vi "FPGAmain_5160.vi"() -> ()   [LabVIEW 2013]
uses:
  FPGA/DataMode.ctl
  FPGA/AcquireState.ctl
  <vilib>/Platform/TimedLoop/XDataNode/timing_clust.ctl
  <vilib>/Platform/TimedLoop/XDataNode/nitl_modes.ctl
  <vilib>/Platform/TimedLoop/XDataNode/wakeup.ctl
  <vilib>/rvi/Emulation/niFpgaSctlEmulationGetInTimedLoop.vi
  <vilib>/rvi/Emulation/niFpgaEmulationReportErrorSimple.vi
  <vilib>/rvi/Emulation/niFpgaGetClockAttributes.vi
  <vilib>/rvi/eio/common/nirviEmuTemplateMethod_errors.vi
  <vilib>/rvi/Emulation/niFpgaCriticalErrorInLSC.vi
  <vilib>/rvi/FIFO/Fifo_Resource/nirvififoEmulationWriteFpgaImpl.vi
  <vilib>/rvi/DataTransferAndStorage/Container/Common/niFpgaContainerGetUniqueNameForEmu.vi
  <vilib>/rvi/FIFO/Fifo_Resource/nirvififoEmulationReadFpgaImpl.vi
  <vilib>/rvi/DataTransferAndStorage/Register/Emulation/niFpgaRegisterEmulationFpgaImpl.vi
  <instcachedir>/0/niFpgaRegisterEmulationFpgaImpl_DCF4BC0110594B98B44A971D60CEEC4D.lvgen/niFpgaRegisterEmulationFpgaImpl_DCF4BC0110594B98B44A971D60CEEC4D_016.vi
  <instcachedir>/0/niFpgaRegisterEmulationFpgaImpl_DCF4BC0110594B98B44A971D60CEEC4D.lvgen/niFpgaRegisterEmulationFpgaImpl_DCF4BC0110594B98B44A971D60CEEC4D_003.vi
  <instcachedir>/0/niFpgaRegisterEmulationFpgaImpl_DCF4BC0110594B98B44A971D60CEEC4D.lvgen/niFpgaRegisterEmulationFpgaImpl_DCF4BC0110594B98B44A971D60CEEC4D_014.vi
  <instcachedir>/0/niFpgaRegisterEmulationFpgaImpl_DCF4BC0110594B98B44A971D60CEEC4D.lvgen/niFpgaRegisterEmulationFpgaImpl_DCF4BC0110594B98B44A971D60CEEC4D_015.vi
  <vilib>/rvi/interface/RandomDataEmulation/nirviRandomDataMultiElementFPGAFIFO.vi
  <instcachedir>/0/nirviRandomDataMultiElementFPGAFIFO_F2B80EDE0D7944A08478D8D26097D4DB.lvgen/nirviRandomDataMultiElementFPGAFIFO_F2B80EDE0D7944A08478D8D26097D4DB_005.vi
  <vilib>/rvi/interface/RandomDataEmulation/niFpgaRandomDataHandleErrors.vi
  <vilib>/rvi/interface/RandomDataEmulation/nirviRandomDataFPGAFIFO.vi
  <vilib>/Platform/TimedLoop/XDataNode/XDataNode.xnode
  <vilib>/eio/EIONode/EIONode.xnode
  <vilib>/rvi/DataTransferAndStorage/Container/XNode/niFpgaContainer.xnode
  <vilib>/rvi/FIFO/Fifo_Resource/nirvififoEmulationWrite.vi
  <vilib>/rvi/FIFO/Fifo_Resource/nirvififoEmulationRead.vi
  <vilib>/rvi/DataTransferAndStorage/Register/Emulation/niFpgaRegisterEmulation.vi
  <vilib>/rvi/interface/RandomDataEmulation/nirviRandomDataFpgaMultiElementTemplate.vi
  <vilib>/rvi/interface/RandomDataEmulation/nirviRandomDataFpgaReadWriteTemplate.vi
  <vilib>/rvi/FIFO/Fifo_Resource/nirvififoEmulationP2P.vi
  <vilib>/Platform/TimedLoop/XDataNode/XDNodeRunTimeDep.lvlib
  <instrlib>/FlexRIO/Libraries/Helper VIs/NI FlexRIO Helper VIs.lvlib
  FPGA/Input_5782/5782_states.ctl
panel:
  in  "delay phase":fxp<+,64,64>
  in  "AM phase":fxp<+,64,64>
  in  "Phase 5782":fxp<+,64,64>[](array[numeric])=[0.0, 0.0]
  in  "User Command Commit":bool
  in  "User Command":u8
  out "User Command Idle":bool
  out "User Command Status":u8
  in  "User Data 0":u8
  in  "User Data 1":u8
  out "PLL Locked":bool
  out "User Error":bool
  out "Configured?":bool
  in  "FIR coeffs":fxp<+/-,18,18>[](array[numeric])
  in  "Phase output":fxp<+,64,64>[](array[numeric])=[0.0, 0.0, 0.0, 0.0]
  in  "5782 record length":u16=4000 caption="Samples Per Trigger" min=1 step=1
  in  "Trigger Acquisition":bool
  in  "Continuous":bool
  out "IO Module\\Trigger Input":bool
  in  "Mode":T1
  in  "Simulated phase 5782":fxp<+,64,64>[](array[numeric])=[0.0, 0.0]
  in  "Acquisition running":bool
  in  "Samples Per Trigger":i32 min=1 step=1
  in  "Trigger simulated data":bool
  in  "simulated phase 5160":fxp<+,64,64>
  in  "phase 5160":fxp<+,64,64>
  # "Dynamic filter"
  # "Dynamic downsample"
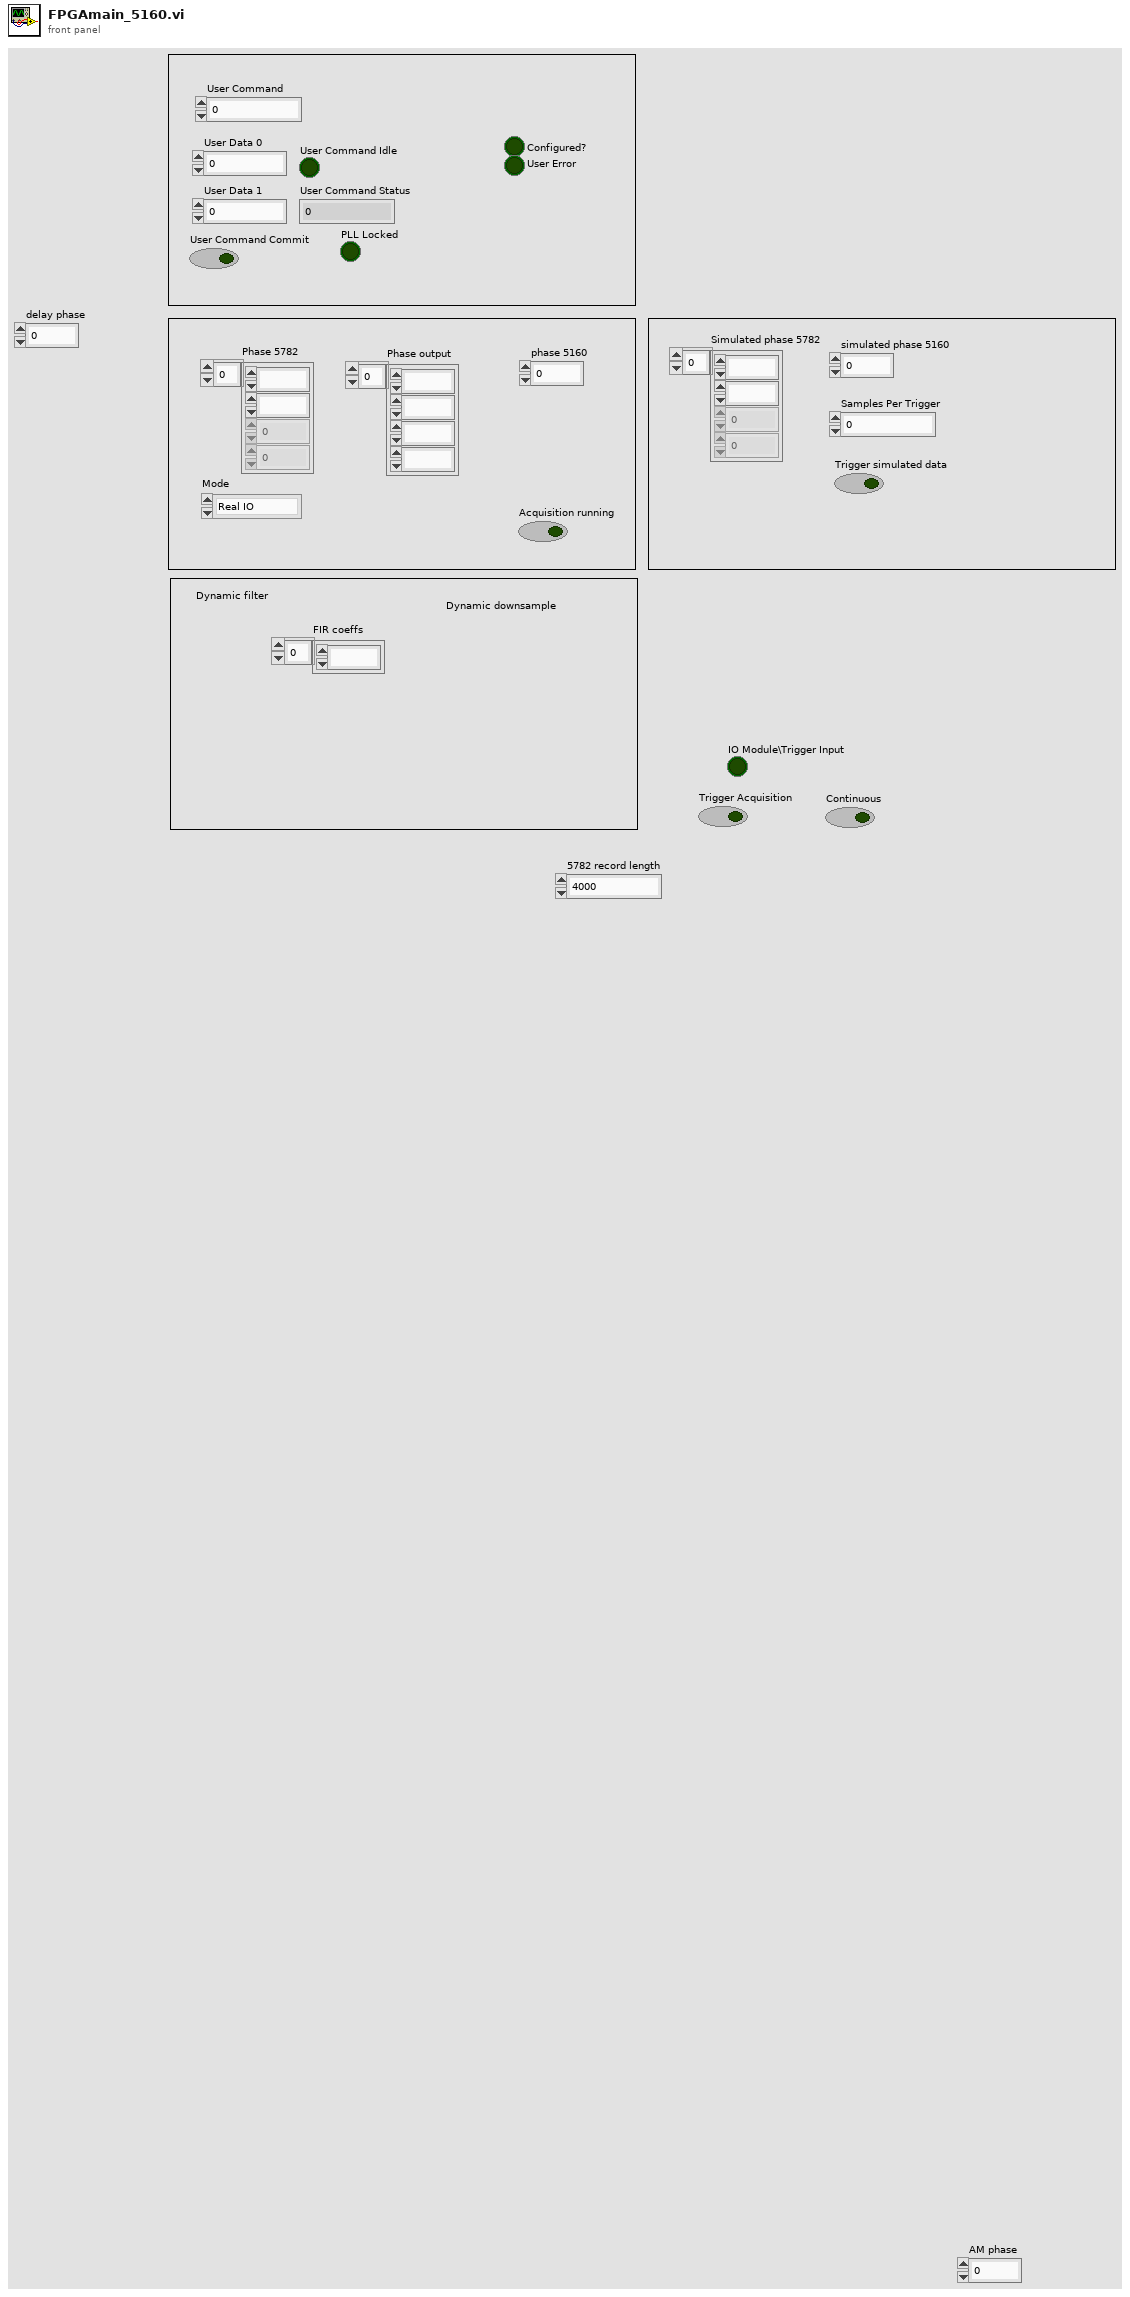
[diagram p1: front panel]
types:
  T1 = typedef "DataMode.ctl" = enum16{"Real IO", "Simulated"}
  T2 = typedef "AcquireState.ctl" = enum8{"Idle", "Acquire"}
  T3 = typedef "5782_states.ctl" = enum8{"Wait for trigger", "Acquisition", "Send record length", "Quiet period"}
  T4 = typedef "XDNodeRunTimeDep.lvlib/timing_clust.ctl" = cluster{"Expected End [f-1]":u64, "Actual End [f-1]":u64, "Finished Late? [f-1]":bool, "Expected End [i-1]":u64, "Actual End [i-1]":u64, "Finished Late? [i-1]":bool, "Expected Start [i]":u64, "Actual Start [i]":u64, "Expected Start [f]":u64, "Actual Start [f]":u64, "Source Name":string, "Structure Name":string, "Period":i64, "Deadline":i64, "Offset":i64, "Start":i64, "Priority":i32, "Timeout":i32, "Mode":T5, "Wakeup Reason":T6, "Error":errorcluster, "Source Type":string, "Secondary Source Type":string, "Global End Time":u64, "Global Start Time":u64, "Frame Duration":u64, "Iteration Duration":u64, "Assigned CPU":i32, "I/O Scan Engine Mode":u32}
  T5 = typedef "XDNodeRunTimeDep.lvlib/nitl_modes.ctl" = enum32{"No Change", "Process missed periods, maintain original phase", "Discard missed periods, maintain original phase", "Process missed periods, ignore original phase", "Discard missed periods, ignore original phase"}
  T6 = typedef "XDNodeRunTimeDep.lvlib/wakeup.ctl" = enum32{"Normal", "Aborted", "Asynchronous wakeup", "Timing source error", "Timed loop error", "Timeout"}
  T7 = typedef "I16 array size 2.ctl" = i16[]
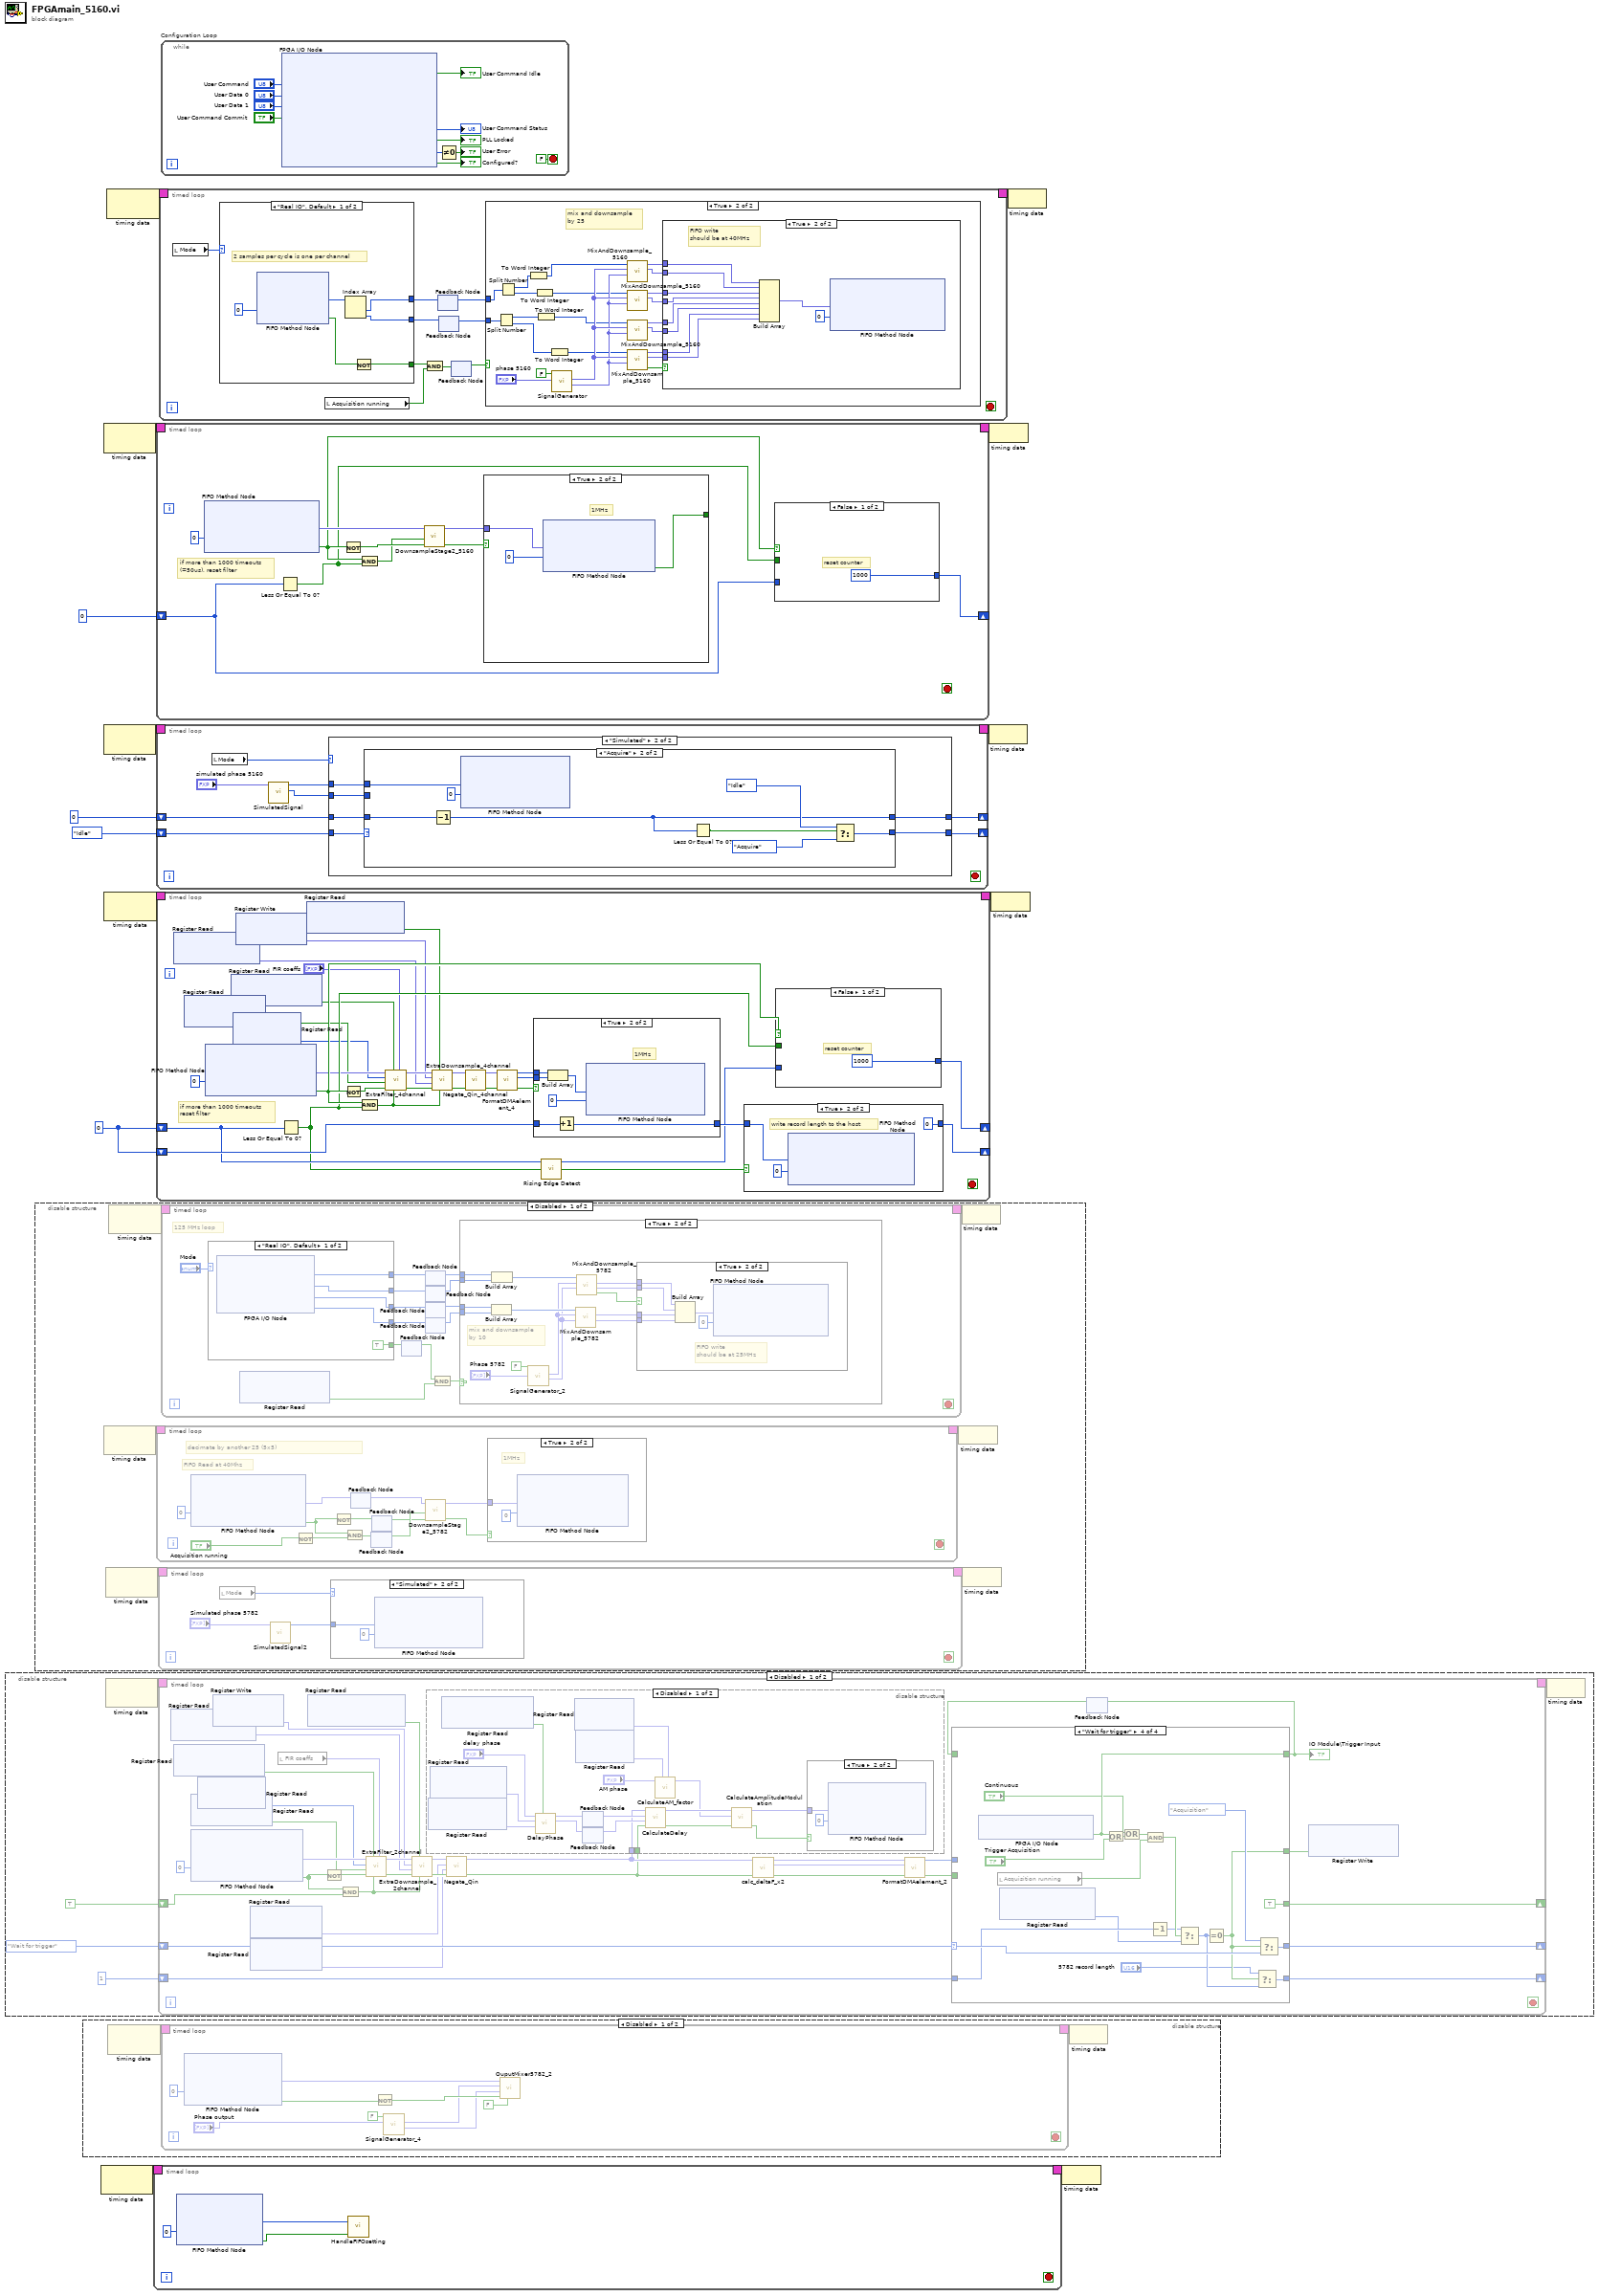
[diagram p0: block diagram]
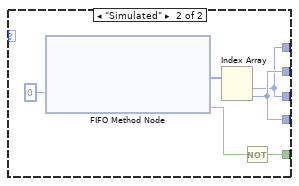
[diagram p4: hidden frame]
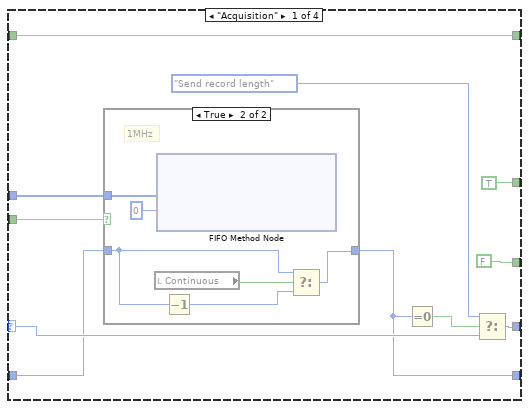
[diagram p10: hidden frame]
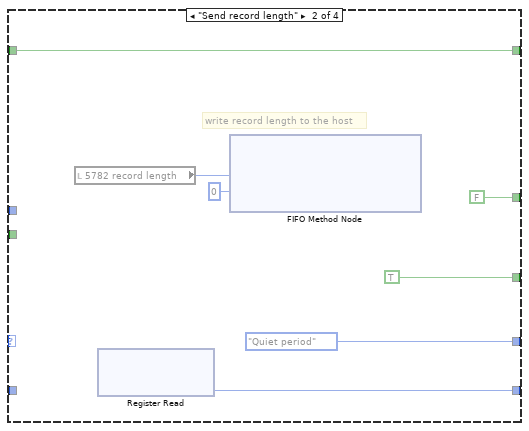
[diagram p12: hidden frame]
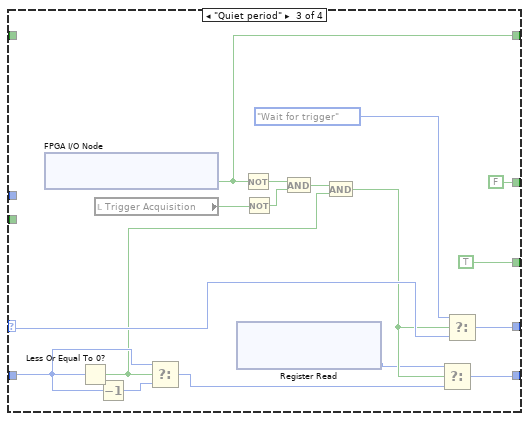
[diagram p13: hidden frame]
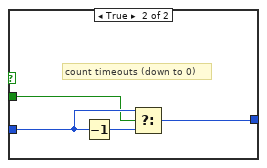
[diagram p16: hidden frame]
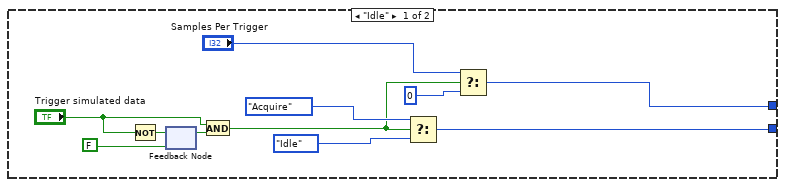
[diagram p20: hidden frame]
diagram:
  w3 = 0 ("y")
  n1 = disable-structure shown="Disabled" {
    frame Disabled {
      n2 = node-c288() -> (w19:T4)  [unwired: 1 in]
      n3 = timed-loop {
        timing: w19 -> [_]
        timing-out: [_] -> w18
        shift-right: [w51] -> _
        shift-left: 5782_states."Wait for trigger" ("5782 states") -> [w53]
        shift-right: [w50] -> _
        shift-left: u16 1 ("trigger samples") -> [w52]
        shift-right: [w39] -> _
        shift-left: TRUE -> [w42]
        stop <- _ stop-if-true
        n4 = xnode ("Register Read")() -> ("Data"=w24:fxp<+,8,8>)  [unwired: 1 in, 1 out]
        n5 = xnode ("Register Read")() -> ("Data"=w30:bool)  [unwired: 1 in, 1 out]
        n6 = xnode ("Register Read")() -> ("Data"=w25:bool)  [unwired: 1 in, 1 out]
        n7 = xnode ("FIFO Method Node")("Timeout"=0) -> ("Element"=w44:fxp<+/-,16,14>[], "Timed Out?"=w43:bool)  [unwired: 1 in, 1 out]
        n8 = xnode ("Register Read")() -> ("Data"=w26:i32)  [unwired: 1 in, 1 out]
        n9 = xnode ("Register Write")() -> ("Data"=w23:fxp<+/-,32,1>)  [unwired: 1 in, 1 out]
        n10 = xnode ("Register Read")() -> ("Data"=w28:fxp<+/-,16,14>)  [unwired: 1 in, 1 out]
        n11 = xnode ("Register Read")() -> ("Data"=w29:fxp<+/-,16,14>)  [unwired: 1 in, 1 out]
        n12 = local read "FIR coeffs"() -> (w22:fxp<+/-,18,18>[])
        n13 = xnode ("Register Read")() -> ("Data"=w27:bool)  [unwired: 1 in, 1 out]
        n14 = Not(x=w43) -> (.not. x?=w46:bool)
        n15 = And(x=w43, y=w42) -> (x .and. y?=w48:bool)
        n16 = call "ExtraFilter_2channel.vi"(5:"new coeffs"=w22, "reset"=w48, 7:"new coeffs"=w30, "valid in"=w46, "enable filter"=w25, "new shift"=w26, "Data in"=w44) -> ("valid out"=w47:bool, "Data out"=w45:fxp<+/-,16,14>[])  [unwired: 3 in]
        n17 = call "ExtraDownsample_2channel.vi"("reset"=w48, "Set downsample"=w27, "valid in"=w47, "Downsample"=w24, "CIC Gain"=w23, "Data in"=w45) -> ("valid out"=w36:bool, "Data out"=w37:fxp<+/-,16,14>[])  [unwired: 4 in]
        n18 = call "Negate_Qin.vi"("valid in"=w36, "DC offset chan 1"=w28, "DC offset chan 0"=w29, "Data in"=w37) -> ("valid out"=w33:bool, "Data out"=w35:fxp<+/-,16,14>[])  [unwired: 6 in]
        n19 = disable-structure shown="Disabled" {
          disable-tunnel: w35 -> [w64 _]
          disable-tunnel: w33 -> [w60 _]
          frame Disabled {
            n20 = xnode ("Register Read")() -> ("Data"=w55:fxp<+/-,16,0>)  [unwired: 1 in, 1 out]
            n21 = xnode ("Register Read")() -> ("Data"=w56:fxp<+/-,16,0>)  [unwired: 1 in, 1 out]
            n22 = xnode ("Register Read")() -> ("Data"=w57:bool)  [unwired: 1 in, 1 out]
            n23 = call "DelayPhase.vi"("Use fixed delay"=w57, "fixed cos_fi"=w55, "fixed sin fi"=w56, "delay phase"="delay phase") -> ("cos_fi"=w62:fxp<+/-,16,0>, "sin fi"=w63:fxp<+/-,16,0>)  [unwired: 6 in]
            n24 = xnode ("Register Read")() -> ("Data"=w59:fxp<+/-,16,2>)  [unwired: 1 in, 1 out]
            n25 = xnode ("Register Read")() -> ("Data"=w58:fxp<+/-,16,2>)  [unwired: 1 in, 1 out]
            n26 = feedback #1() -> (w71:fxp<+/-,16,0>)  [unwired: 1 in]
            n27 = feedback-in #1(w63) -> ()
            n28 = feedback #2() -> (w70:fxp<+/-,16,0>)  [unwired: 1 in]
            n29 = feedback-in #2(w62) -> ()
            n30 = call "CalculateDelay.vi"("input valid"=w60, "cos_fi"=w70, "sin fi"=w71, "Data in"=w64) -> ("output valid"=w68:bool, "Data out"=w69:fxp<+/-,16,14>[])  [unwired: 6 in]
            n31 = call "CalculateAM_factor.vi"("b_am"=w59, "a_am"=w58, "AM phase"="AM phase") -> ("AM_factor"=w65:fxp<+/-,16,2>)  [unwired: 7 in, 1 out]
            n32 = call "CalculateAmplitudeModulation.vi"("input valid"=w68, "AM_factor"=w65, "Data in"=w69) -> ("output valid"=w66:bool, "Data out"=w67:fxp<+/-,16,14>[])  [unwired: 7 in]
            n33 = case shown="True" w66 {
              tunnel: w67 -> [_ w72]
              frame False {
              }
              frame True {
                n34 = xnode ("FIFO Method Node")("Element"=w72, "Timeout"=0) -> ()  [unwired: 1 in, 2 out]
              }
            }
          }
          frame Enabled {
          }
        }
        n35 = call "calc_deltaF_x2.vi"("valid in"=w33, "Data in"=w35) -> ("valid out"=w32:bool, "deltaF"=w31:fxp<+/-,32,30>[], "Data out"=w34:fxp<+/-,16,14>[])  [unwired: 7 in]
        n36 = call "FormatDMAelement_2.vi"("valid in"=w32, "deltaF"=w31, "Data in"=w34) -> ("valid out"=w40:bool, "Element"=w41:u64[])  [unwired: 7 in]
        n37 = feedback #3() -> (w21:bool)  [unwired: 1 in]
        n38 = case shown="\"Wait for trigger\"" w53 {
          selector: w53 -> [w84 _ w114 w133]
          tunnel: w52 -> [w80 _ w102 w122]
          tunnel: [w83 5782_states."Quiet period" ("5782 states") w113 w132] -> w51
          tunnel: [w77 w92 w115 w131] -> w50
          tunnel: w41 -> [w78 _ _ _]
          tunnel: w40 -> [w79 _ _ _]
          tunnel: [FALSE TRUE TRUE TRUE] -> w39
          tunnel: [TRUE FALSE ("5782 triggered") FALSE ("5782 triggered") w126] -> w38
          tunnel: [w76 w93 w104 w125] -> w20
          tunnel: w21 -> [w76 w93 _ _]
          frame "Acquisition" {
            n39 = case shown="True" w79 {
              tunnel: w78 -> [_ w91]
              tunnel: [w85 w88] -> w77
              tunnel: w80 -> [w85 w86]
              frame False {
              }
              frame True {
                # "1MHz"
                n40 = local read "Continuous"() -> (w89:bool)
                n41 = xnode ("FIFO Method Node")("Element"=w91, "Timeout"=0) -> ()  [unwired: 1 in, 2 out]
                n42 = Decrement(x=w86) -> (x-1=w87:u16)
                n43 = Select(t=w86, s=w89, f=w87) -> (s? t:f=w88:u16)
              }
            }
            n44 = Equal To 0?(x=w77) -> (x = 0?=w81:bool)
            n45 = Select(t=5782_states."Send record length" ("5782 states"), s=w81, f=w84) -> (s? t:f=w83:T3)
          }
          frame "Send record length" {
            # "write record length to the host"
            n46 = local read "5782 record length"() -> (w95:u16)
            n47 = xnode ("Register Read")() -> ("Data"=w92:u16)  [unwired: 1 in, 1 out]
            n48 = xnode ("FIFO Method Node")("Element"=w95, "Timeout"=0) -> ()  [unwired: 1 in, 2 out]
          }
          frame "Quiet period" {
            n49 = xnode "FPGA I/O Node"() -> ("IO Module\\Trigger Input"=w104:bool)  [unwired: 1 in, 1 out]
            n50 = Less Or Equal To 0?(x=w102) -> (x <= 0?=w101:bool)
            n51 = local read "Trigger Acquisition"() -> (w110:bool)
            n52 = Decrement(x=w102) -> (x-1=w103:u16)
            n53 = Select(t=w102, s=w101, f=w103) -> (s? t:f=w100:u16)
            n54 = xnode ("Register Read")() -> ("Data"=w99:u16)  [unwired: 1 in, 1 out]
            n55 = Not(x=w104) -> (.not. x?=w109:bool)
            n56 = Not(x=w110) -> (.not. x?=w108:bool)
            n57 = And(x=w109, y=w108) -> (x .and. y?=w107:bool)
            n58 = And(x=w107, y=w101) -> (x .and. y?=w112:bool)
            n59 = Select(t=w99, s=w112, f=w100) -> (s? t:f=w115:u16)
            n60 = Select(t=5782_states."Wait for trigger" ("5782 states"), s=w112, f=w114) -> (s? t:f=w113:T3)
          }
          frame "Wait for trigger" {
            n61 = xnode "FPGA I/O Node"() -> ("IO Module\\Trigger Input"=w125:bool)  [unwired: 1 in, 1 out]
            n62 = local read "Acquisition running"() -> (w127:bool)
            n63 = xnode ("Register Read")() -> ("Data"=w119:u16)  [unwired: 1 in, 1 out]
            n64 = Or(x=w125, y="Trigger Acquisition") -> (x .or. y?=w121:bool)
            n65 = Or(x="Continuous", y=w121) -> (x .or. y?=w120:bool)
            n66 = And(x=w120, y=w127) -> (x .and. y?=w128:bool)
            n67 = Decrement(x=w122) -> (x-1=w123:u16)
            n68 = Select(t=w123, s=w128, f=w119) -> (s? t:f=w124:u16)
            n69 = Equal To 0?(x=w124) -> (x = 0?=w126:bool)
            n70 = Select(t="5782 record length", s=w126, f=w124) -> (s? t:f=w131:u16)
            n71 = Select(t=5782_states."Acquisition" ("5782 states"), s=w126, f=w133) -> (s? t:f=w132:T3)
          }
        }
        "IO Module\\Trigger Input" <- w20
        n72 = feedback-in #3(w20) -> ()
        n73 = xnode ("Register Write")("Data"=w38) -> ()  [unwired: 1 in, 1 out]
      }
      n74 = node-c288(w18) -> ()
    }
    frame Enabled {
    }
  }
  n75 = disable-structure shown="Disabled" {
    frame Disabled {
      n76 = node-c288() -> (w141:T4)  [unwired: 1 in]
      n77 = node-c288() -> (w143:T4)  [unwired: 1 in]
      n78 = node-c288() -> (w139:T4)  [unwired: 1 in]
      n79 = timed-loop {
        timing: w141 -> [_]
        timing-out: [_] -> w140
        stop <- _ stop-if-true
        # "FIFO Read at 40Mhz"
        # "decimate by another 25 (5x5)"
        n80 = xnode ("FIFO Method Node")("Timeout"=0) -> ("Element"=w199:fxp<+/-,16,14>[], "Timed Out?"=w200:bool)  [unwired: 1 in, 1 out]
        n81 = Not(x="Acquisition running") -> (.not. x?=w201:bool)
        n82 = Not(x=w200) -> (.not. x?=w195:bool)
        n83 = And(x=w200, y=w201) -> (x .and. y?=w197:bool)
        n84 = feedback #4() -> (w198:fxp<+/-,16,14>[])  [unwired: 1 in]
        n85 = feedback-in #4(w199) -> ()
        n86 = feedback #5() -> (w196:bool)  [unwired: 1 in]
        n87 = feedback-in #5(w197) -> ()
        n88 = feedback #6() -> (w194:bool)  [unwired: 1 in]
        n89 = feedback-in #6(w195) -> ()
        n90 = call "DownsampleStage2_5782.vi"("valid in"=w194, "reset"=w196, "Data in"=w198) -> ("valid out"=w202:bool, "data out"=w203:fxp<+/-,16,14>[])  [unwired: 7 in]
        n91 = case shown="True" w202 {
          tunnel: w203 -> [_ w205]
          frame False {
          }
          frame True {
            # "1MHz"
            n92 = xnode ("FIFO Method Node")("Element"=w205, "Timeout"=0) -> ()  [unwired: 1 in, 2 out]
          }
        }
      }
      n93 = timed-loop {
        timing: w143 -> [_]
        timing-out: [_] -> w142
        stop <- _ stop-if-true
        n94 = local read "Mode"() -> (w213:T1)
        n95 = call "SimulatedSignal2.vi"("Phase"="Simulated phase 5782") -> ("output"=w212:T7)  [unwired: 9 in, 1 out]
        n96 = case shown="\"Simulated\"" w213 {
          tunnel: w212 -> [_ w214]
          frame "Real IO", Default {
          }
          frame "Simulated" {
            n97 = xnode ("FIFO Method Node")("Element"=w214, "Timeout"=0) -> ()  [unwired: 1 in, 2 out]
          }
        }
      }
      n98 = timed-loop {
        timing: w139 -> [_]
        timing-out: [_] -> w138
        stop <- _ stop-if-true
        # "125 MHz loop"
        n99 = case shown="\"Real IO\", Default" "Mode" {
          tunnel: [w182 w185] -> w155
          tunnel: [w181 w186] -> w153
          tunnel: [w180 w185] -> w151
          tunnel: [w179 w186] -> w148
          tunnel: [TRUE w183] -> w147
          frame "Real IO", Default {
            n100 = xnode "FPGA I/O Node"() -> ("IO Module\\AI 0 N-1"=w182:i16, "IO Module\\AI 0 N"=w181:i16, "IO Module\\AI 1 N-1"=w180:i16, "IO Module\\AI 1 N"=w179:i16)  [unwired: 4 in, 4 out]
          }
          frame "Simulated" {
            n101 = xnode ("FIFO Method Node")("Timeout"=0) -> ("Element"=w187:i16[], "Timed Out?"=w184:bool)  [unwired: 1 in, 1 out]
            n102 = Index Array(array=w187) -> (element #1=w185:i16, element #2=w186:i16)  [unwired: 2 in]
            n103 = Not(x=w184) -> (.not. x?=w183:bool)
          }
        }
        n104 = xnode ("Register Read")() -> ("Data"=w145:bool)  [unwired: 1 in, 1 out]
        n105 = feedback #7() -> (w146:bool)  [unwired: 1 in]
        n106 = feedback-in #7(w147) -> ()
        n107 = feedback #8() -> (w154:i16)  [unwired: 1 in]
        n108 = feedback-in #8(w155) -> ()
        n109 = feedback #9() -> (w152:i16)  [unwired: 1 in]
        n110 = feedback-in #9(w153) -> ()
        n111 = feedback #10() -> (w150:i16)  [unwired: 1 in]
        n112 = feedback-in #10(w151) -> ()
        n113 = feedback #11() -> (w149:i16)  [unwired: 1 in]
        n114 = feedback-in #11(w148) -> ()
        n115 = And(x=w146, y=w145) -> (x .and. y?=w156:bool)
        n116 = case shown="True" w156 {
          tunnel: w154 -> [_ w162]
          tunnel: w152 -> [_ w161]
          tunnel: w150 -> [_ w160]
          tunnel: w149 -> [_ w159]
          frame False {
          }
          frame True {
            # "mix and downsample\nby 10"
            n117 = Build Array(w160, w159) -> (w171:i16[])
            n118 = Build Array(w162, w161) -> (w158:i16[])
            n119 = call "SignalGenerator_2.vi"("Phase"="Phase 5782", "reset"=FALSE) -> ("Sine out"=w163:fxp<+/-,16,0>[], "Cosine out"=w164:fxp<+/-,16,0>[])  [unwired: 8 in]
            n120 = call "MixAndDownsample_5782.vi"("Sine in"=w163, "Cosine in"=w164, "Signal Input"=w171) -> ("Q out"=w166:fxp<+/-,16,14>, "I out"=w167:fxp<+/-,16,14>)  [unwired: 6 in, 1 out]
            n121 = call "MixAndDownsample_5782.vi"("Sine in"=w163, "Cosine in"=w164, "Signal Input"=w158) -> ("data valid"=w168:bool, "Q out"=w169:fxp<+/-,16,14>, "I out"=w170:fxp<+/-,16,14>)  [unwired: 6 in]
            n122 = case shown="True" w168 {
              tunnel: w169 -> [_ w177]
              tunnel: w170 -> [_ w174]
              tunnel: w167 -> [_ w173]
              tunnel: w166 -> [_ w172]
              frame False {
              }
              frame True {
                # "FIFO write\nshould be at 25MHz"
                n123 = Build Array(w174, w177, w173, w172) -> (w176:fxp<+/-,16,14>[])
                n124 = xnode ("FIFO Method Node")("Element"=w176, "Timeout"=0) -> ()  [unwired: 1 in, 2 out]
              }
            }
          }
        }
      }
      n125 = node-c288(w140) -> ()
      n126 = node-c288(w138) -> ()
      n127 = node-c288(w142) -> ()
    }
    frame Enabled {
    }
  }
  n128 = disable-structure shown="Disabled" {
    frame Disabled {
      n129 = node-c288() -> (w221:T4)  [unwired: 1 in]
      n130 = timed-loop {
        timing: w221 -> [_]
        timing-out: [_] -> w220
        stop <- _ stop-if-true
        n131 = xnode ("FIFO Method Node")("Timeout"=0) -> ("Element"=w222:fxp<+/-,16,14>[], "Timed Out?"=w224:bool)  [unwired: 1 in, 1 out]
        n132 = Not(x=w224) -> (.not. x?=w228:bool)
        n133 = call "SignalGenerator_4.vi"("Phase"="Phase output", "reset"=FALSE) -> ("Sine out"=w225:fxp<+/-,16,0>[], "Cosine out"=w226:fxp<+/-,16,0>[])  [unwired: 8 in]
        n134 = call "OuputMixer5782_2.vi"("reset"=FALSE, "valid in"=w228, "Sine in"=w225, "Cosine in"=w226, "Data in"=w222) -> ()  [unwired: 5 in, 2 out]
      }
      n135 = node-c288(w220) -> ()
    }
    frame Enabled {
    }
  }
  n136 = node-c288() -> (w2:T4)  [unwired: 1 in]
  n137 = node-c288() -> (w12:T4)  [unwired: 1 in]
  n138 = node-c288() -> (w10:T4)  [unwired: 1 in]
  n139 = node-c288() -> (w5:T4)  [unwired: 1 in]
  n140 = node-c288() -> (w14:T4)  [unwired: 1 in]
  n141 = timed-loop {
    timing: w2 -> [_]
    timing-out: [_] -> w1
    stop <- _ stop-if-true
    n142 = xnode ("FIFO Method Node")("Timeout"=0) -> ("Element"=w236:u64, "Timed Out?"=w235:bool)  [unwired: 1 in, 1 out]
    n143 = call "HandleFIFOsetting.vi"("timed out"=w235, "Value"=w236) -> ()  [unwired: 10 in]
  }
  n144 = timed-loop {
    timing: w12 -> [_]
    timing-out: [_] -> w11
    shift-right: [w242] -> _
    shift-left: 0 ("y") -> [w241]
    stop <- _ stop-if-true
    # "if more than 1000 timeouts\n(=50us), reset filter"
    n145 = xnode ("FIFO Method Node")("Timeout"=0) -> ("Element"=w246:fxp<+/-,16,14>[], "Timed Out?"=w243:bool)  [unwired: 1 in, 1 out]
    n146 = Less Or Equal To 0?(x=w241) -> (x <= 0?=w240:bool)
    n147 = Not(x=w243) -> (.not. x?=w247:bool)
    n148 = And(x=w243, y=w240) -> (x .and. y?=w244:bool)
    n149 = call "DownsampleStage2_5160.vi"("valid in"=w247, "reset"=w244, "Element"=w246) -> ("valid out"=w248:bool, "Array"=w249:fxp<+/-,16,14>[])  [unwired: 7 in]
    n150 = case shown="True" w248 {
      tunnel: w249 -> [_ w256]
      tunnel: [FALSE ("Timed Out?") w257] -> _
      frame False {
      }
      frame True {
        # "1MHz"
        n151 = xnode ("FIFO Method Node")("Element"=w256, "Timeout"=0) -> ("Timed Out?"=w257:bool)  [unwired: 1 in, 1 out]
      }
    }
    n152 = case shown="False" w243 {
      tunnel: w240 -> [_ w252]
      tunnel: w241 -> [_ w253]
      tunnel: [1000 ("y") w251] -> w242
      frame False {
        # "reset counter"
      }
      frame True {
        # "count timeouts (down to 0)"
        n153 = Decrement(x=w253) -> (x-1=w254:i32)
        n154 = Select(t=w253, s=w252, f=w254) -> (s? t:f=w251:i32)
      }
    }
  }
  n155 = timed-loop {
    timing: w10 -> [_]
    timing-out: [_] -> w9
    shift-right: [w264] -> _
    shift-left: 0 ("f") -> [w263]
    shift-right: [w262] -> _
    shift-left: AcquireState."Idle" ("Acquire State") -> [w261]
    stop <- _ stop-if-true
    n156 = local read "Mode"() -> (w268:T1)
    n157 = call "SimulatedSignal.vi"("phase"="simulated phase 5160") -> ("cos output"=w266:i16, "Sample output"=w267:i16)  [unwired: 9 in]
    n158 = case shown="\"Simulated\"" w268 {
      tunnel: w267 -> [_ w276]
      tunnel: w266 -> [_ w271]
      tunnel: [w270 w275] -> w264
      tunnel: w263 -> [w270 w274]
      tunnel: [w269 w273] -> w262
      tunnel: w261 -> [w269 w272]
      frame "Real IO" {
      }
      frame "Simulated" {
        n159 = case shown="\"Acquire\"" w272 {
          tunnel: w274 -> [_ w292]
          tunnel: [w281 w291] -> w273
          tunnel: [w278 w290] -> w275
          tunnel: w276 -> [_ w289]
          tunnel: w271 -> [_ _]
          frame "Idle" {
            n160 = Not(x="Trigger simulated data") -> (.not. x?=w282:bool)
            n161 = feedback #12(FALSE) -> (w283:bool)
            n162 = feedback-in #12(w282) -> ()
            n163 = And(x="Trigger simulated data", y=w283) -> (x .and. y?=w277:bool)
            n164 = Select(t=AcquireState."Acquire" ("Acquire State"), s=w277, f=AcquireState."Idle" ("Acquire State")) -> (s? t:f=w281:T2)
            n165 = Select(t="Samples Per Trigger", s=w277, f=0) -> (s? t:f=w278:i32)
          }
          frame "Acquire" {
            n166 = Decrement(x=w292) -> (x-1=w290:i32)
            n167 = xnode ("FIFO Method Node")("Element"=w289, "Timeout"=0) -> ()  [unwired: 1 in, 2 out]
            n168 = Less Or Equal To 0?(x=w290) -> (x <= 0?=w294:bool)
            n169 = Select(t=AcquireState."Idle" ("Acquire State"), s=w294, f=AcquireState."Acquire" ("Acquire State")) -> (s? t:f=w291:T2)
          }
        }
      }
    }
  }
  n170 = timed-loop {
    timing: w5 -> [_]
    timing-out: [_] -> w4
    shift-right: [w320] -> _
    shift-left: w3 -> [w319]
    shift-right: [w322] -> _
    shift-left: w3 -> [w324]
    stop <- _ stop-if-true
    # "if more than 1000 timeouts\nreset filter"
    n171 = xnode ("Register Read")() -> ("Data"=w301:fxp<+,8,8>)  [unwired: 1 in, 1 out]
    n172 = xnode ("Register Read")() -> ("Data"=w299:bool)  [unwired: 1 in, 1 out]
    n173 = xnode ("FIFO Method Node")("Timeout"=0) -> ("Element"=w315:fxp<+/-,16,14>[], "Timed Out?"=w321:bool)  [unwired: 1 in, 1 out]
    n174 = xnode ("Register Read")() -> ("Data"=w300:bool)  [unwired: 1 in, 1 out]
    n175 = xnode ("Register Read")() -> ("Data"=w298:i32)  [unwired: 1 in, 1 out]
    n176 = xnode ("Register Write")() -> ("Data"=w302:fxp<+/-,32,1>)  [unwired: 1 in, 1 out]
    n177 = Less Or Equal To 0?(x=w319) -> (x <= 0?=w318:bool)
    n178 = xnode ("Register Read")() -> ("Data"=w303:bool)  [unwired: 1 in, 1 out]
    n179 = Not(x=w321) -> (.not. x?=w314:bool)
    n180 = And(x=w321, y=w318) -> (x .and. y?=w316:bool)
    n181 = call "ExtraFilter_4channel.vi"(5:"new coeffs"="FIR coeffs", "reset"=w316, 7:"new coeffs"=w300, "valid in"=w314, "enable filter"=w299, "new shift"=w298, "Data in"=w315) -> ("valid out"=w305:bool, "Data out"=w306:fxp<+/-,16,14>[])  [unwired: 3 in]
    n182 = call "ExtraDownsample_4channel.vi"("reset"=w316, "Set downsample"=w303, "valid in"=w305, "Downsample"=w301, "CIC Gain"=w302, "Data in"=w306) -> ("valid out"=w307:bool, "Data out"=w310:fxp<+/-,16,14>[])  [unwired: 4 in]
    n183 = call "Negate_Qin_4channel.vi"("valid in"=w307, "Data in"=w310) -> ("valid out"=w308:bool, "Data out"=w309:fxp<+/-,16,14>[])  [unwired: 8 in]
    n184 = call "FormatDMAelement_4.vi"("valid in"=w308, "Data in"=w309) -> ("valid out"=w311:bool, "Element2"=w312:u64, "Element1"=w313:u64)  [unwired: 7 in]
    n185 = case shown="True" w311 {
      tunnel: w313 -> [_ w340]
      tunnel: w312 -> [_ w339]
      tunnel: w324 -> [w335 w337]
      tunnel: [w335 w336] -> w323
      frame False {
      }
      frame True {
        # "1MHz"
        n186 = Build Array(w340, w339) -> (w338:u64[])
        n187 = Increment(x=w337) -> (x+1=w336:i32)
        n188 = xnode ("FIFO Method Node")("Element"=w338, "Timeout"=0) -> ()  [unwired: 1 in, 2 out]
      }
    }
    n189 = call <instrlib>:"Rising Edge Detect.vi"("signal"=w318) -> ("edge detected"=w317:bool)  [unwired: 14 in]
    n190 = case shown="True" w317 {
      tunnel: w323 -> [w331 w332]
      tunnel: [w331 0 ("y")] -> w322
      frame False {
      }
      frame True {
        # "write record length to the host"
        n191 = xnode ("FIFO Method Node")("Element"=w332, "Timeout"=0) -> ()  [unwired: 1 in, 2 out]
      }
    }
    n192 = case shown="False" w321 {
      tunnel: w318 -> [_ w328]
      tunnel: w319 -> [_ w329]
      tunnel: [1000 ("y") w327] -> w320
      frame False {
        # "reset counter"
      }
      frame True {
        # "count timeouts (down to 0)"
        n193 = Decrement(x=w329) -> (x-1=w330:i32)
        n194 = Select(t=w329, s=w328, f=w330) -> (s? t:f=w327:i32)
      }
    }
  }
  n195 = timed-loop {
    timing: w14 -> [_]
    timing-out: [_] -> w13
    stop <- _ stop-if-true
    n196 = local read "Mode"() -> (w347:T1)
    n197 = case shown="\"Real IO\", Default" w347 {
      tunnel: [w389 w395] -> w352
      tunnel: [w386 w392] -> w346
      tunnel: [w388 w395] -> w349
      frame "Real IO", Default {
        # "2 samples per cycle is one per channel"
        n198 = xnode ("FIFO Method Node")("Timeout"=0) -> ("Element"=w391:u32[], "Timed Out?"=w387:bool)  [unwired: 1 in, 1 out]
        n199 = Index Array(array=w391) -> (element #1=w389:u32, element #2=w388:u32)  [unwired: 2 in]
        n200 = Not(x=w387) -> (.not. x?=w386:bool)
      }
      frame "Simulated" {
        n201 = xnode ("FIFO Method Node")("Timeout"=0) -> ("Element"=w394:i16, "Timed Out?"=w393:bool)  [unwired: 1 in, 1 out]
        n202 = Not(x=w393) -> (.not. x?=w392:bool)
        n203 = Join Numbers(hi=w394, lo=w394) -> ((hi.lo)=w395:u32)
      }
    }
    n204 = local read "Acquisition running"() -> (w345:bool)
    n205 = And(x=w346, y=w345) -> (x .and. y?=w344:bool)
    n206 = feedback-in #13(w352) -> ()
    n207 = feedback #13() -> (w351:u32)  [unwired: 1 in]
    n208 = feedback #14() -> (w348:u32)  [unwired: 1 in]
    n209 = feedback-in #14(w349) -> ()
    n210 = feedback #15() -> (w350:bool)  [unwired: 1 in]
    n211 = feedback-in #15(w344) -> ()
    n212 = case shown="True" w350 {
      tunnel: w351 -> [_ w366]
      tunnel: w348 -> [_ w355]
      frame False {
        # "FIFO read timeout, no data"
      }
      frame True {
        # "mix and downsample\nby 25"
        n213 = Split Number(x=w355) -> (hi(x)=w356:u16, lo(x)=w357:u16)
        n214 = Split Number(x=w366) -> (hi(x)=w365:u16, lo(x)=w364:u16)
        n215 = To Word Integer(number=w365) -> (16bit integer=w359:i16)
        n216 = To Word Integer(number=w364) -> (16bit integer=w358:i16)
        n217 = To Word Integer(number=w356) -> (16bit integer=w353:i16)
        n218 = To Word Integer(number=w357) -> (16bit integer=w354:i16)
        n219 = call "SignalGenerator.vi"("phase"="phase 5160", "Reset"=FALSE) -> ("Cos"=w360:fxp<+/-,16,0>, "Sin"=w361:fxp<+/-,16,0>)  [unwired: 7 in, 1 out]
        n220 = call "MixAndDownsample_5160.vi"("Sine in"=w360, "Cosine in"=w361, "Sample in"=w359) -> ("Q out"=w373:fxp<+/-,16,14>, "I out"=w375:fxp<+/-,16,14>)  [unwired: 6 in, 1 out]
        n221 = call "MixAndDownsample_5160.vi"("Sine in"=w360, "Cosine in"=w361, "Sample in"=w358) -> ("Q out"=w371:fxp<+/-,16,14>, "I out"=w372:fxp<+/-,16,14>)  [unwired: 6 in, 1 out]
        n222 = call "MixAndDownsample_5160.vi"("Sine in"=w360, "Cosine in"=w361, "Sample in"=w353) -> ("Q out"=w369:fxp<+/-,16,14>, "I out"=w370:fxp<+/-,16,14>)  [unwired: 6 in, 1 out]
        n223 = call "MixAndDownsample_5160.vi"("Sine in"=w360, "Cosine in"=w361, "Sample in"=w354) -> ("valid out"=w374:bool, "Q out"=w367:fxp<+/-,16,14>, "I out"=w368:fxp<+/-,16,14>)  [unwired: 6 in]
        n224 = case shown="True" w374 {
          tunnel: w375 -> [_ w384]
          tunnel: w373 -> [_ w383]
          tunnel: w372 -> [_ w382]
          tunnel: w371 -> [_ w376]
          tunnel: w370 -> [_ w381]
          tunnel: w369 -> [_ w380]
          tunnel: w368 -> [_ w379]
          tunnel: w367 -> [_ w378]
          frame False {
          }
          frame True {
            # "FIFO write\nshould be at 40MHz"
            n225 = Build Array(w384, w383, w382, w376, w381, w380, w379, w378) -> (w377:fxp<+/-,16,14>[])
            n226 = xnode ("FIFO Method Node")("Element"=w377, "Timeout"=0) -> ()  [unwired: 1 in, 2 out]
          }
        }
      }
    }
  }
  n227 = while "Configuration Loop" {
    stop <- FALSE stop-if-true
    n228 = xnode "FPGA I/O Node"("IO Module\\User Command"="User Command", "IO Module\\User Data 0"="User Data 0", "IO Module\\User Data 1"="User Data 1", "IO Module\\User Command Commit"="User Command Commit") -> ("IO Module\\User Command Idle"=→"User Command Idle":bool, "IO Module\\User Command Status"=→"User Command Status":u8, "IO Module\\PLL Locked"=→"PLL Locked":bool, "IO Module\\User Error"=w404:u8, "IO Module\\Initialization Done"=→"Configured?":bool)  [unwired: 9 in, 9 out]
    n229 = Not Equal To 0?(x=w404) -> (x != 0?=→"User Error":bool)
  }
  n230 = node-c288(w9) -> ()
  n231 = node-c288(w11) -> ()
  n232 = node-c288(w4) -> ()
  n233 = node-c288(w13) -> ()
  n234 = node-c288(w1) -> ()
